vi "Dnamic resizing testing.vi"() -> ()   [LabVIEW 2014]
panel:
  in  "Width":i16
  in  "Height":i16
  in  "Left":i16
  in  "Top":i16
  in  "stop":bool
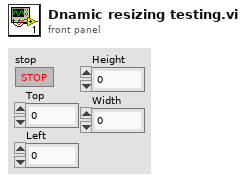
[diagram p1: front panel]
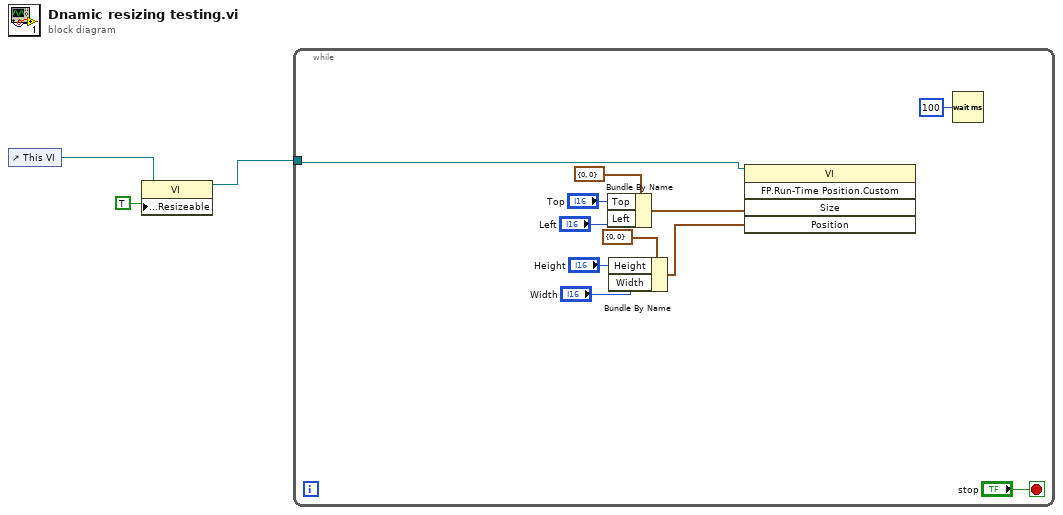
[diagram p0: block diagram]
diagram:
  n1 = control-ref of="This VI"() -> (w3:refnum<vi>)
  n2 = property class="VI"(reference=w3, "Front Panel.Resizeable"=TRUE ("Front Panel Window:Resizable")) -> (reference out=w2:refnum<vi>)  [unwired: 1 in, 1 out]
  n3 = while {
    tunnel: w2 -> [w12]
    stop <- "stop" stop-if-true
    n4 = Bundle By Name(cluster=cluster{"Top":i16, "Left":i16} {"Top"=0, "Left"=0} ("Position"), "Top"="Top", "Left"="Left") -> (w10:cluster{"Top":i16, "Left":i16})
    n5 = Bundle By Name(cluster=cluster{"Height":i16, "Width":i16} {"Height"=0, "Width"=0} ("Size"), "Height"="Height", "Width"="Width") -> (w6:cluster{"Height":i16, "Width":i16})
    n6 = invoke class="VI" method="FP.Run-Time Position.Custom"(reference=w12, "Size"=w10, "Position"=w6) -> ()  [unwired: 2 in, 5 out]
    n7 = Wait (ms)(milliseconds to wait=u32 100) -> ()  [unwired: 1 out]
  }
